vi "Read channels.vi"(8 "error in (no error)":errorcluster, 11 "RT State Data in":T1) -> (0 "error out":errorcluster, 3 "RT State Data out":T1)   [LabVIEW 2013, in "Waveforms Generation Custom Device.lvlib"]
uses:
  Waveforms Generation Custom Device.lvlib
  RT state data.ctl
  <vilib>/NI Veristand/Custom Device Waveform API/Multiple Waveforms Write (DBL)/Multiple Waveforms Write (DBL).lvclass
  <vilib>/NI Veristand/Custom Device API/Waveform Data Reference.ctl
  <vilib>/NI Veristand/Custom Device API/Custom Device API.lvlib
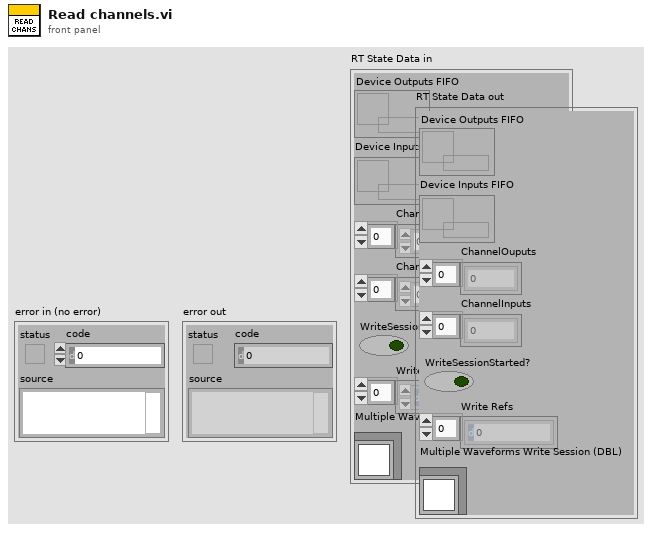
[diagram p1: front panel]
types:
  T1 = typedef "Waveforms Generation Custom Device.lvlib/RT state data.ctl" = cluster{"Device Outputs FIFO":refnum<k33>, "Device Inputs FIFO":refnum<k33>, "ChannelOuputs":dbl[], "ChannelInputs":dbl[], "WriteSessionStarted?":bool, "Write Refs":T2[], "Multiple Waveforms Write Session (DBL)":refnum<class "Multiple Waveforms Write (DBL).lvclass">}
  T2 = typedef "Custom Device API.lvlib/Waveform Data Reference.ctl" = i32
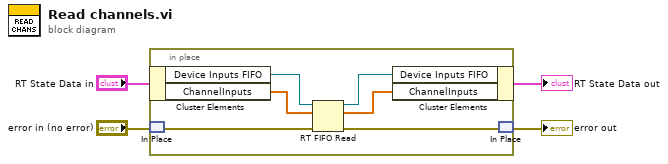
[diagram p0: block diagram]
diagram:
  n1 = in-place {
    n2 = in-place-cluster #1("RT State Data in") -> ("Device Inputs FIFO"=w8:refnum<k33>, "ChannelInputs"=w9:dbl[])
    n3 = in-place-match #2("error in (no error)") -> (w10:errorcluster)
    n4 = RT FIFO Read(0:w8, 1:w9, 3:w10) -> (8:w7:refnum<k33>, 9:w6:dbl[], 11:w5:errorcluster)  [unwired: 3 out]
    n5 = in-place-cluster #1("Device Inputs FIFO"=w7, "ChannelInputs"=w6) -> (→"RT State Data out":T1)
    n6 = in-place-match #2(w5) -> (→"error out":errorcluster)
  }
